vi "PAS_set_channel.vi"(8 "error in (no error)":errorcluster, 10 "Channel":u16(ring) items=["DAC", "ADC 1 (temp)", "ADC 2", "ADC 3"], 11 "VISA Refnum in":refnum<visa-resource-name>) -> (0 "error out":errorcluster, 1 "Success?":bool, 3 "VISA Refnum out":refnum<visa-resource-name>)   [LabVIEW 2020]
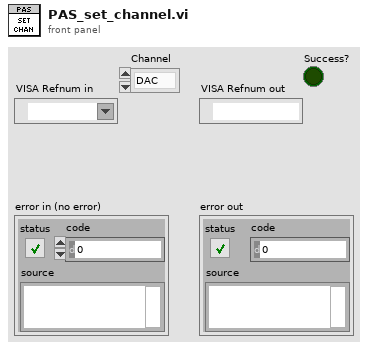
[diagram p1: front panel]
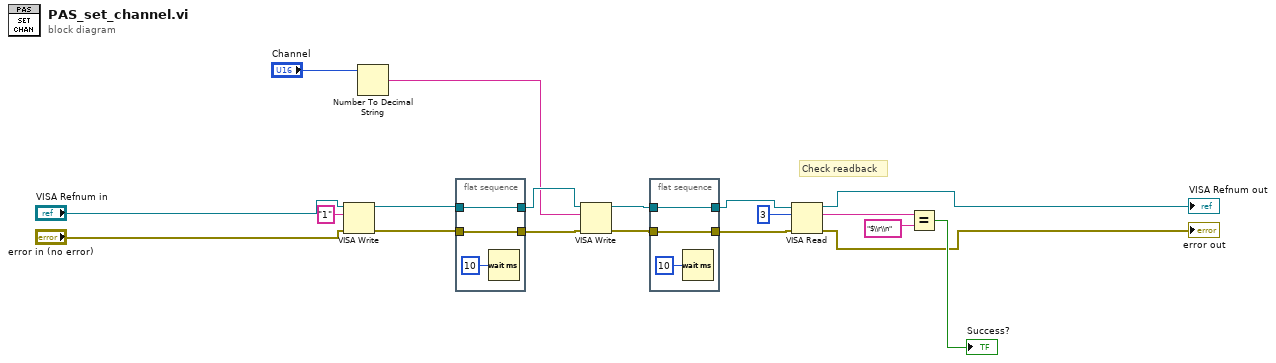
[diagram p0: block diagram]
diagram:
  # "Check readback"
  n1 = VISA Write(VISA resource name="VISA Refnum in", write buffer="1", error in (no error)="error in (no error)") -> (VISA resource name out=w14:refnum<visa-resource-name>, error out=w15:errorcluster)  [unwired: 1 out]
  n2 = Number To Decimal String(number="Channel") -> (decimal integer string=w11:string)  [unwired: 1 in]
  n3 = flat-sequence {
    tunnel: w14 -> [w21]
    tunnel: [w21] -> w16
    tunnel: w15 -> [w20]
    tunnel: [w20] -> w17
    frame #0 {
      n4 = Wait (ms)(milliseconds to wait=u32 10) -> ()  [unwired: 1 out]
    }
  }
  n5 = VISA Write(VISA resource name=w16, write buffer=w11, error in (no error)=w17) -> (VISA resource name out=w2:refnum<visa-resource-name>, error out=w4:errorcluster)  [unwired: 1 out]
  n6 = flat-sequence {
    tunnel: w2 -> [w24]
    tunnel: [w24] -> w1
    tunnel: w4 -> [w23]
    tunnel: [w23] -> w3
    frame #0 {
      n7 = Wait (ms)(milliseconds to wait=u32 10) -> ()  [unwired: 1 out]
    }
  }
  n8 = VISA Read(VISA resource name=w1, byte count=u32 3, error in (no error)=w3) -> (VISA resource name out=→"VISA Refnum out":refnum<visa-resource-name>, read buffer=w9:string, error out=→"error out":errorcluster)  [unwired: 1 out]
  n9 = Equal?(x=w9, y="$\\r\\n") -> (x = y?=→"Success?":bool)
